vi "SimpleUART.vi"() -> ()   [LabVIEW 2019]
uses:
  <userlib>/MicroPython/VIs/uPythonX/uPythonX.xctl
panel:
  in  "Simple":T1(xcontrol)={"Port"="HighPeaksPYBD - ASRL114::INSTR", "All Code"="import machine, utime, gc\n\nuart = machine.UART(1)\nuart.init(baudrate=9600, bits=8, parity=None, stop=1)\n\nwhile True:\n     if uart.any():\n          chr = uart.readchar()\n          print(chr)\n          fred=bytearray([chr])\n          print (fred)\n          sent = uart.write(fred)\n"}
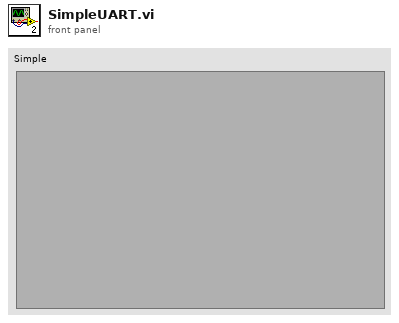
[diagram p1: front panel]
types:
  T1 = cluster{"Port":refnum<visa-resource-name>, "All Code":string}
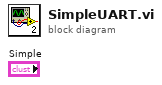
[diagram p0: block diagram]
diagram:
